vi "Append or Replace 2D Array Element (I8).vi"(6 "Default":i8, 8 "Element":i8, 9 "Indices (>=1D)":i32[](array[numeric]), 10 "Index (1D)":i32, 11 "Array In":i8[][](array[numeric])) -> (3 "Array Out":i8[][](array[numeric]))   [LabVIEW 2009]
doc: "Appends or replaces the array element at given indices. Inefficient for large arrays."
panel:
  # "Append or Replace Array Element.vi\n\nAppends or replaces the array element at given indices.  Inefficient for large arrays.  Currently implemented only for 1D and 2D arrays.\n\nPlease visit http://www.OpenG.org to learn about the\nOpen Source LabVIEW software movement.\n\nNOTICE -- YOU MUST LEAVE THIS NOTICE IN PLACE.  PER THE TERMS OF THE LICENSE BELOW, YOU MAY SUBLICENSE THIS SOFTWARE \nIN ANY WAY THAT DOES NOT CONFLICT WITH THIS LICENSE.\n\n### BSD License (http://www.opensource.org/licenses/bsd-license.php) Begin ###\n \nCopyright (c) 2005, MKS Instruments, Inc., author: Doug Femec<doug_femec@mksinst.com>, IM dafemec\n\nAll rights reserved.\n\nRedistribution and use in source and binary forms, with or without modification, are permitted provided that the following conditions are met:\n\n    * Redistributions of source code must retain the above copyright notice, this list of conditions and the following disclaimer.\n    * Redistributions in binary form must reproduce the above copyright notice, this list of conditions and the following disclaimer in the \n       documentation and/or other materials provided with the distribution.\n    * Neither the name of SciWare, James Kring, Inc., nor the names of its contributors may be used to endorse or promote products derived \n       from this software without specific prior written permission.\n\nTHIS SOFTWARE IS PROVIDED BY THE COPYRIGHT HOLDERS AND CONTRIBUTORS \"AS IS\" AND ANY EXPRESS OR IMPLIED WARRANTIES, \nINCLUDING, BUT NOT LIMITED TO, THE IMPLIED WARRANTIES OF MERCHANTABILITY AND FITNESS FOR A PARTICULAR PURPOSE ARE \nDISCLAIMED. IN NO EVENT SHALL THE COPYRIGHT OWNER OR CONTRIBUTORS BE LIABLE FOR ANY DIRECT, INDIRECT, INCIDENTAL,\n SPECIAL, EXEMPLARY, OR CONSEQUENTIAL DAMAGES (INCLUDING, BUT NOT LIMITED TO, PROCUREMENT OF SUBSTITUTE GOODS OR \nSERVICES; LOSS OF USE, DATA, OR PROFITS; OR BUSINESS INTERRUPTION) HOWEVER CAUSED AND ON ANY THEORY OF LIABILITY, \nWHETHER IN CONTRACT, STRICT LIABILITY, OR TORT (INCLUDING NEGLIGENCE OR OTHERWISE) ARISING IN ANY WAY OUT OF THE USE \nOF THIS SOFTWARE, EVEN IF ADVISED OF THE POSSIBILITY OF SUCH DAMAGE.\n\n### BSD License End ###"
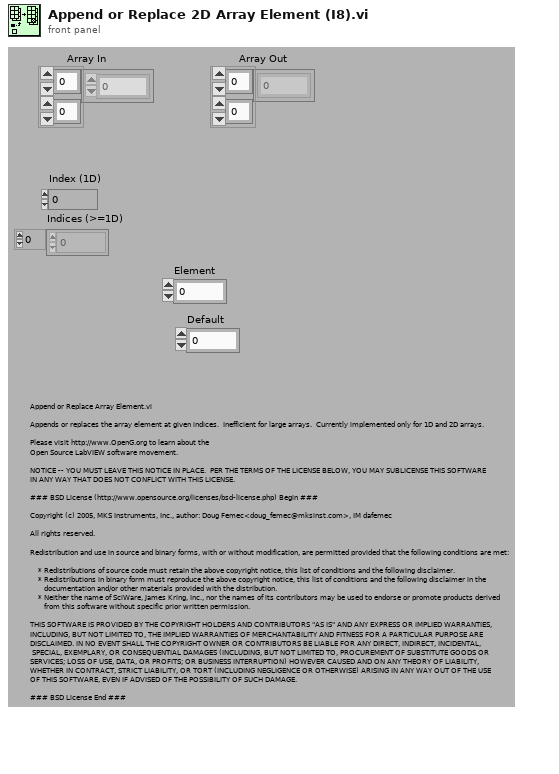
[diagram p1: front panel]
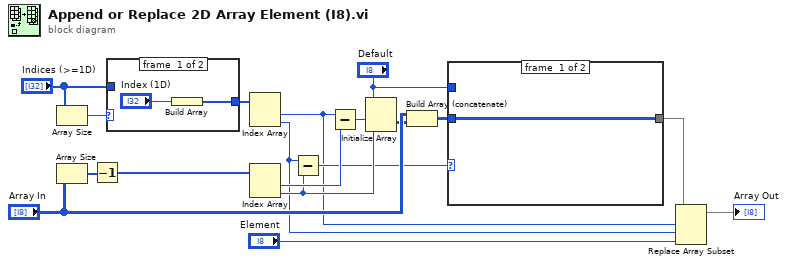
[diagram p0: block diagram]
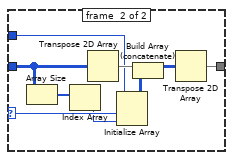
[diagram p2: hidden frame]
diagram:
  n1 = Array Size(array="Indices (>=1D)") -> (size(s)=w16:i32)
  n2 = Array Size(array="Array In") -> (size(s)=w13:i32[])
  n3 = Decrement(x=w13) -> (x-1=w12:i32[])
  n4 = case shown="0" w16 {
    tunnel: [w19 w21] -> w14
    tunnel: "Indices (>=1D)" -> [_ w21]
    frame #0 {
      n5 = Build Array("Index (1D)") -> (w19:i32[])
    }
    frame #1 {
    }
  }
  n6 = Index Array(array=w14) -> (element #1=w1:i32, element #2=w2:i32)  [unwired: 2 in]
  n7 = Index Array(array=w12) -> (element #1=w11:i32, element #2=w6:i32)  [unwired: 2 in]
  n8 = Subtract(x=w2, y=w6) -> (x-y=w3:i32)
  n9 = Subtract(x=w1, y=w11) -> (x-y=w10:i32)
  n10 = Initialize Array("Default", w10, w6) -> (w9:i8[][])
  n11 = Build Array (concatenate)("Array In", w9) -> (w8:i8[][])
  n12 = case shown="1.." w3 {
    selector: w3 -> [_ w26]
    tunnel: w8 -> [w22 w25]
    tunnel: [w22 w31] -> w5
    tunnel: "Default" -> [_ w27]
    frame #0 {
    }
    frame #1 {
      n13 = Array Size(array=w25) -> (size(s)=w24:i32[])
      n14 = Index Array(array=w24) -> (element=w23:i32)  [unwired: 1 in]
      n15 = Transpose 2D Array(2D array=w25) -> (transposed array=w30:i8[][])
      n16 = Initialize Array(w27, w26, w23) -> (w28:i8[][])
      n17 = Build Array (concatenate)(w30, w28) -> (w29:i8[][])
      n18 = Transpose 2D Array(2D array=w29) -> (transposed array=w31:i8[][])
    }
  }
  n19 = Replace Array Subset(array=w5, new element="Element", index (row)=w1, index (col)=w2) -> (→"Array Out":i8[][])
